vi "FlyWheelSim_SetInput.vi"(9 "Battery_Volts":dbl=12.0, 10 "Volts":dbl, 11 "FlyWheelSim":T1 {"GearBox"."Kt_NMPerAmp" format="%13.5p"; "GearBox"."Kv_RadPerSecPerVolt" format="%13.5p"; "GearBox"."R_Ohms" format="%13.5p"; "GearBox"."FreeSpeed_RadPerSec" format="%13.5p"; "GearBox"."FreeCurrent_Amps" format="%13.5p"; "GearBox"."StallCurrent_Amps" format="%13.5p"; "GearBox"."StallTorque_NM" format="%13.5p"; "GearBox"."nominalVoltage_Volts" format="%13.5p"}) -> (3 "out FlyWheelSim":T1 {"GearBox"."Kt_NMPerAmp" format="%13.5p"; "GearBox"."Kv_RadPerSecPerVolt" format="%13.5p"; "GearBox"."R_Ohms" format="%13.5p"; "GearBox"."FreeSpeed_RadPerSec" format="%13.5p"; "GearBox"."FreeCurrent_Amps" format="%13.5p"; "GearBox"."StallCurrent_Amps" format="%13.5p"; "GearBox"."StallTorque_NM" format="%13.5p"; "GearBox"."nominalVoltage_Volts" format="%13.5p"})   [LabVIEW 2019, in "Trajectory_Library.lvlib"]
doc: "Creates a new LINEAR SYSTEM data cluster with the specified values. \n\n\nInputs: \n - XXX -- XXX.\n\nOutputs:\n - XXX -- XXX."
uses:
  Trajectory_Library.lvlib
  FLYWHEEL_SIM.ctl
  LINEAR_SYSTEM_SIM.ctl
  LINEAR_SYSTEM.ctl
  <vilib>/Analysis/Matrix/Datatypes/RealMatrix.ctl
  DCMOTOR.CTL
  <vilib>/Analysis/Matrix/NI_Matrix.lvlib
panel:
  # "<States, 1>"
  # "<Outputs, 1>"
  # "<Inputs, 1>"
  # "<Outputs, 1>"
  # "<States,States>"
  # "<States,Inputs>"
  # "<Outputs,States>"
  # "<Outputs,Inputs>"
  # "<States, 1>"
  # "<Outputs, 1>"
  # "<Inputs, 1>"
  # "<Outputs, 1>"
  # "<States,States>"
  # "<States,Inputs>"
  # "<Outputs,States>"
  # "<Outputs,Inputs>"
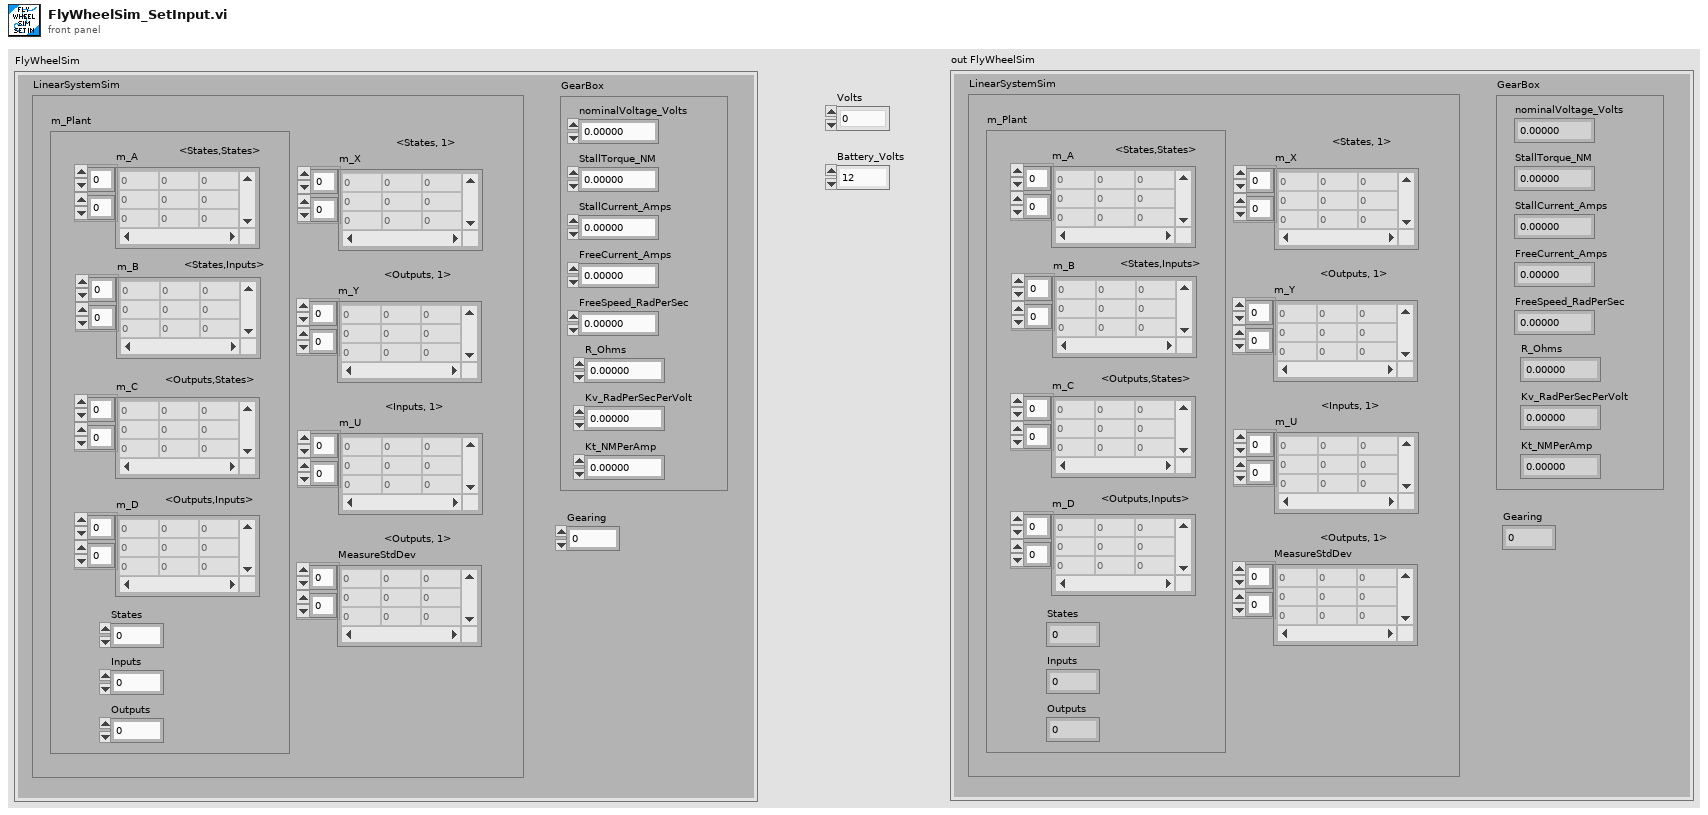
[diagram p1: front panel]
types:
  T1 = typedef "Trajectory_Library.lvlib/FLYWHEEL_SIM.ctl" = cluster{"LinearSystemSim":T2, "GearBox":T5, "Gearing":dbl}
  T2 = typedef "Trajectory_Library.lvlib/LINEAR_SYSTEM_SIM.ctl" = cluster{"m_Plant":T3, "m_X":T4, "m_Y":T4, "m_U":T4, "MeasureStdDev":T4}
  T3 = typedef "Trajectory_Library.lvlib/LINEAR_SYSTEM.ctl" = cluster{"m_A":T4, "m_B":T4, "m_C":T4, "m_D":T4, "States":i32, "Inputs":i32, "Outputs":i32}
  T4 = typedef "NI_Matrix.lvlib/RealMatrix.ctl" = dbl[][]
  T5 = typedef "Trajectory_Library.lvlib/DCMOTOR.CTL" = cluster{"nominalVoltage_Volts":dbl, "StallTorque_NM":dbl, "StallCurrent_Amps":dbl, "FreeCurrent_Amps":dbl, "FreeSpeed_RadPerSec":dbl, "R_Ohms":dbl, "Kv_RadPerSecPerVolt":dbl, "Kt_NMPerAmp":dbl}
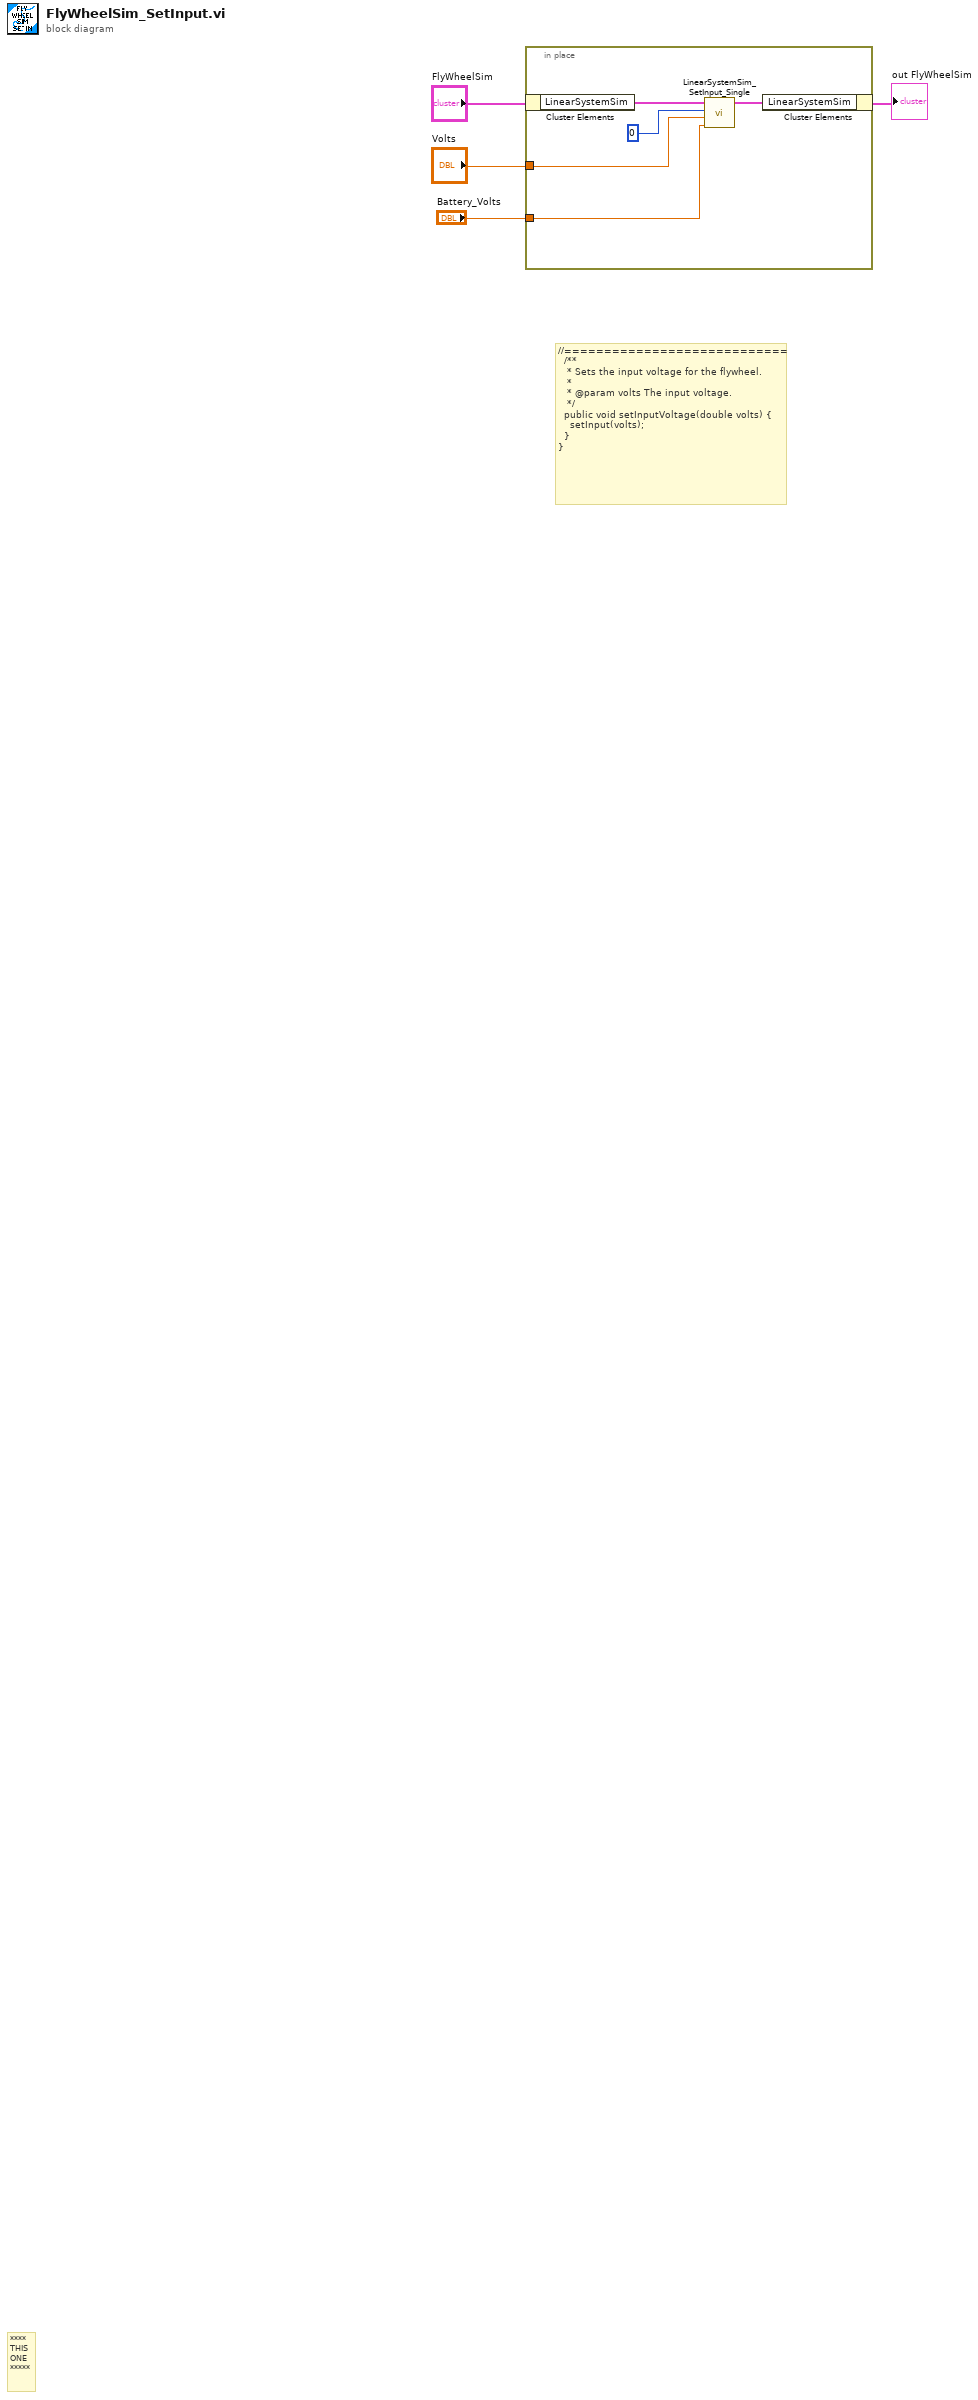
[diagram p0: block diagram]
diagram:
  # "//============================\n  /**\n   * Sets the input voltage for the flywheel.\n   *\n   * @param volts The input voltage.\n   */\n  public void setInputVoltage(double volts) {\n    setInput(volts);\n  }\n}"
  # "****\nTHIS\nONE\n*****"
  n1 = in-place {
    in-place-border: "Volts" -> [w6]
    in-place-border: "Battery_Volts" -> [w5]
    n2 = in-place-cluster #1("FlyWheelSim") -> ("LinearSystemSim"=w9:T2)
    n3 = call "LinearSystemSim_SetInput_Single.vi"("Battery_Volts"=w5, "Input Value"=w6, "Row"=0, "in LinearSystemSim"=w9) -> ("out LinearSystemSim"=w8:T2)  [unwired: 7 in]
    n4 = in-place-cluster #1("LinearSystemSim"=w8) -> (→"out FlyWheelSim":T1)
  }
